vi "Validate_RegGroups.vi"(8 "error in (no error)":errorcluster, 11 "IB_MSI in":refnum<class "IB_MSI.lvclass">) -> (0 "error out":errorcluster, 3 "IB_MSI out":refnum<class "IB_MSI.lvclass">)   [LabVIEW 2020, in "IB_MSI.lvclass"]
uses:
  <vilib>/AppBuilder/IB_Classes/MSI/IB_MSI.lvclass
  <vilib>/AppBuilder/IB_Classes/MSI/IB_MSI.lvclass/IB_MSI.ctl
  <vilib>/AppBuilder/IB_Classes/RegDest/IB_RegDest.lvclass
  <vilib>/AppBuilder/IB_Classes/RegGroup/IB_RegGroup.lvclass
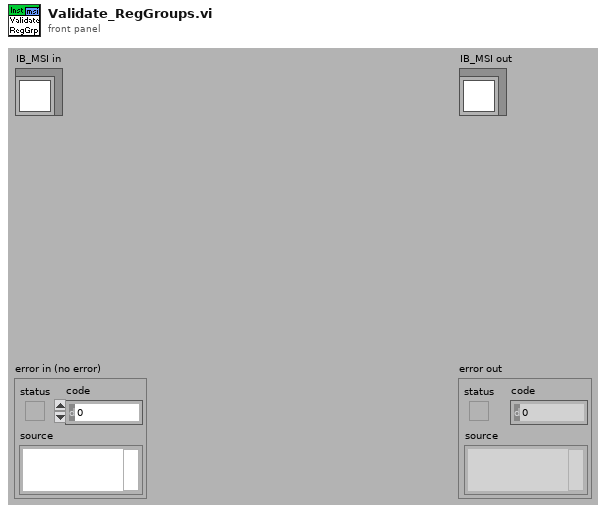
[diagram p1: front panel]
types:
  T1 = typedef "IB_RegDest.ctl" = cluster{"parentTag":string, "dirTag":string, "dirName":string, "unlock":bool, "path":string, "regData":refnum<class "IB_RegData.lvclass">[]}
  T2 = typedef "IB_RegGroup.ctl" = cluster{"RegData":refnum<class "IB_RegData.lvclass">[], "dirTag":string}
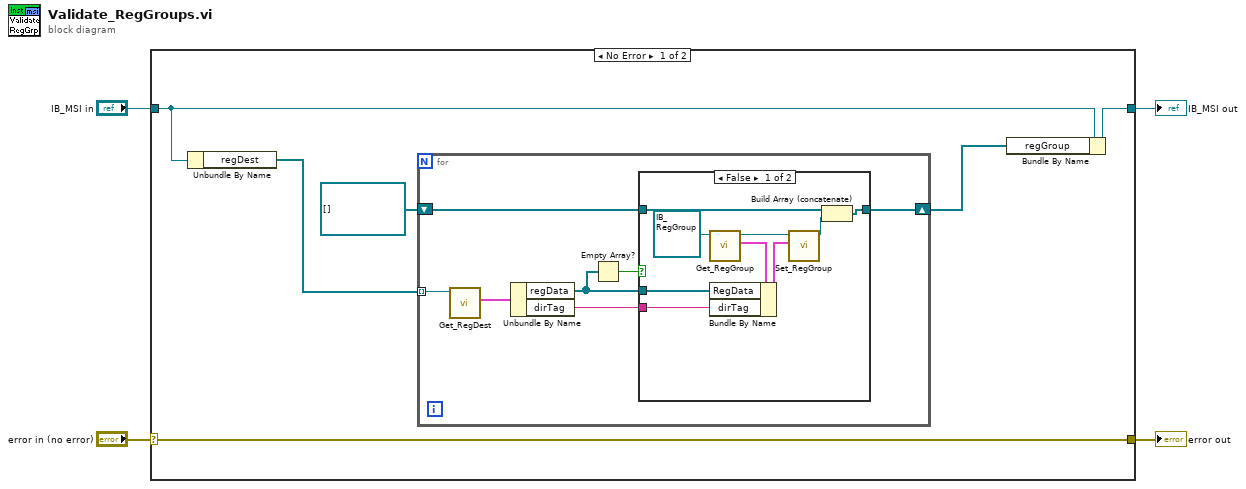
[diagram p0: block diagram]
diagram:
  n1 = case shown="No Error" "error in (no error)" {
    selector: "error in (no error)" -> [w10 w29]
    tunnel: [w10 w29] -> w3
    tunnel: [w7 w28] -> w1
    tunnel: "IB_MSI in" -> [w8 w28]
    frame No Error {
      n2 = Unbundle By Name(w8) -> ("regDest"=w9:refnum<class "IB_RegDest.lvclass">[])
      n3 = for {
        tunnel: w9 -> [w17] mode=indexing
        shift-right: [w11] -> w5
        shift-left: refnum<class "IB_RegGroup.lvclass">[] [] -> [w12]
        n4 = call <vilib>:"Get_RegDest.vi"("Class in"=w17) -> ("data"=w16:T1)  [unwired: 1 in, 9 out]
        n5 = Unbundle By Name(w16) -> ("regData"=w14:refnum<class "IB_RegData.lvclass">[], "dirTag"=w13:string)
        n6 = Empty Array?(array=w14) -> (empty?=w15:bool)
        n7 = case shown="False" w15 {
          tunnel: w14 -> [w22 _]
          tunnel: w13 -> [w21 _]
          tunnel: w12 -> [w20 w27]
          tunnel: [w18 w27] -> w11
          frame False {
            n8 = call <vilib>:"Get_RegGroup.vi"("IB_RegGroup in"=refnum<class "IB_RegGroup.lvclass"> refnum ("IB_RegGroup.lvclass")) -> ("data"=w24:T2, "IB_RegGroup out"=w25:refnum<class "IB_RegGroup.lvclass">)  [unwired: 1 in, 8 out]
            n9 = Bundle By Name(cluster=w24, "RegData"=w22, "dirTag"=w21) -> (w23:T2)
            n10 = call <vilib>:"Set_RegGroup.vi"("data"=w23, "IB_RegGroup in"=w25) -> ("IB_RegGroup out"=w19:refnum<class "IB_RegGroup.lvclass">)  [unwired: 1 in, 8 out]
            n11 = Build Array (concatenate)(w20, w19) -> (w18:refnum<class "IB_RegGroup.lvclass">[])
          }
          frame True {
          }
        }
      }
      n12 = Bundle By Name(cluster=w8, "regGroup"=w5) -> (w7:refnum<class "IB_MSI.lvclass">)
    }
    frame Error {
    }
  }
  "error out" <- w3
  "IB_MSI out" <- w1
